vi "myCommClose.vi"(8 "错误输入（无错误）":errorcluster, 10 "地址":u16, 11 "Modbus Master输入":refnum<class "Modbus Master.lvclass">) -> ()   [LabVIEW 2024]
uses:
  <vilib>/NI/Modbus Library/API/Master/Modbus Master.lvclass
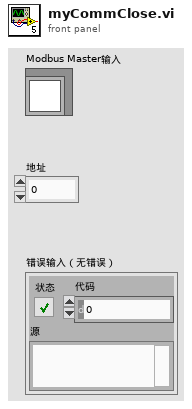
[diagram p1: front panel]
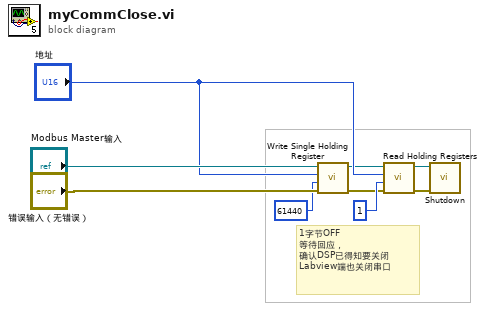
[diagram p0: block diagram]
diagram:
  # "1字节OFF\n等待回应，\n确认DSP已得知要关闭\nLabview端也关闭串口"
  n1 = call-dynamic "Write Single Holding Register.vi"("error in"="错误输入（无错误）", "register to write"=u16 61440, "address"="地址", "Modbus master in"="Modbus Master输入") -> ("error out"=w2:errorcluster, "Modbus master out"=w3:refnum<class "Modbus Master.lvclass">)  [unwired: 6 in]
  n2 = call-dynamic "Read Holding Registers.vi"("error in"=w2, "number of inputs"=u16 1, "starting address"="地址", "Modbus master in"=w3) -> ("error out"=w5:errorcluster, "Modbus master out"=w4:refnum<class "Modbus Master.lvclass">)  [unwired: 5 in, 1 out]
  n3 = call-dynamic "Shutdown.vi"("error in"=w5, "Modbus master in"=w4) -> ()  [unwired: 9 in, 1 out]
